vi "AutoTuneLockin.vi"() -> ()   [LabVIEW 2011]
panel:
  out "LockinXrange":dbl
  out "SlideY":cluster{dbl, dbl}(slide)={0.0, -1.6336633663366336} scale=-1.0..1.0
  out "Slide 2":cluster{dbl, dbl}(slide)={0.0, -1.6336633663366336} scale=-1.0..1.0
  out "Y":dbl
  out "X":dbl
  in  "stop":bool
  in  "Lockin":refnum<visa-resource-name>
  in  "Sr 830 sensitivity":T1(ring)
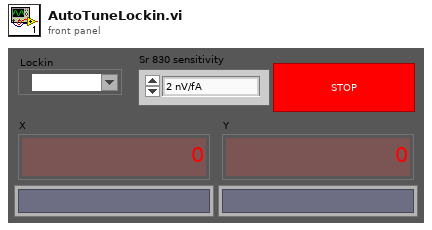
[diagram p1: front panel]
types:
  T1 = enum16{"2 nV/fA", "5 nV/fA", "10 nV/fA", "20 nV/fA", "50 nV/fA", "100 nV/fA", "200 nV/fA", "500 nV/fA", "1 uV/pA", "2 uV/pA", "5 uV/pA", "10 uV/pA", "20 uV/pA", "50 uV/pA", "100 uV/pA", "200 uV/pA", "500 uV/pA", "1 mV/nA", "2 mV/nA", "5 mV/nA", "10 mV/nA", "20 mV/nA", "50 mV/nA", "100 mV/nA", "200 mV/nA", "500 mV/nA", "1 V/uA"}
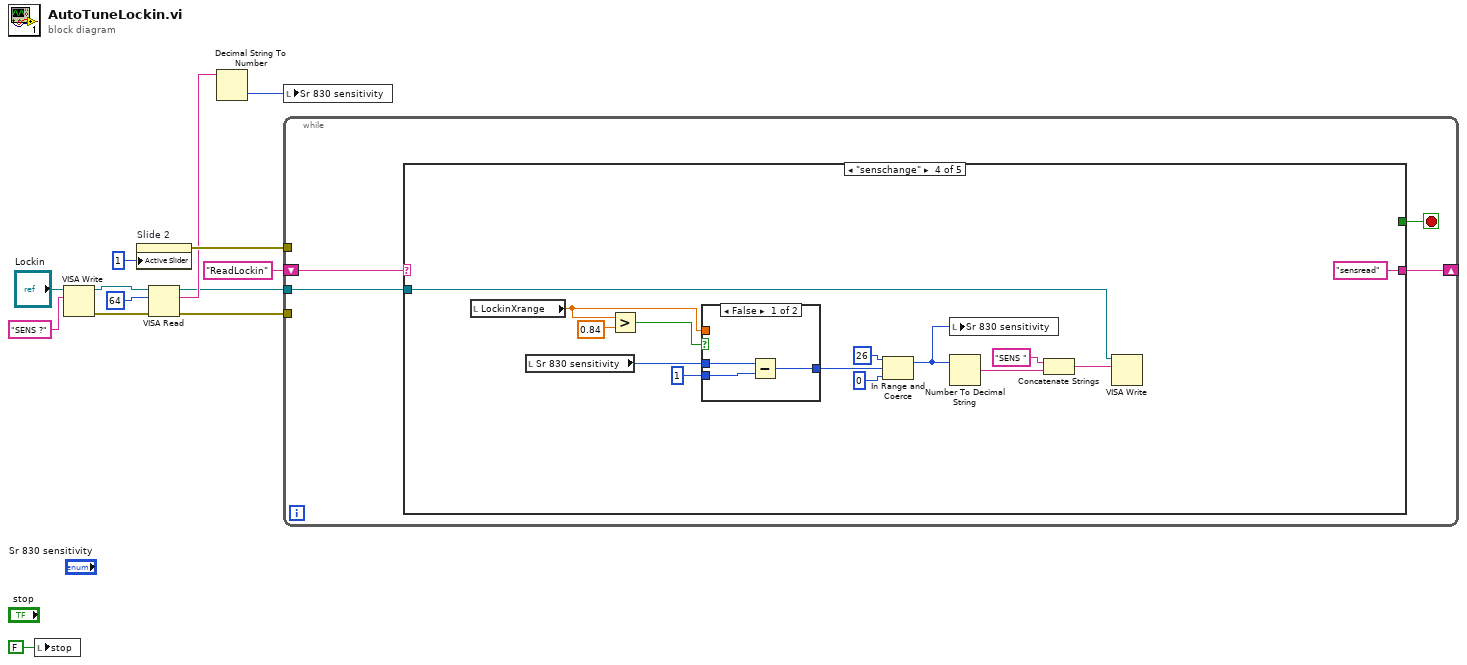
[diagram p0: block diagram]
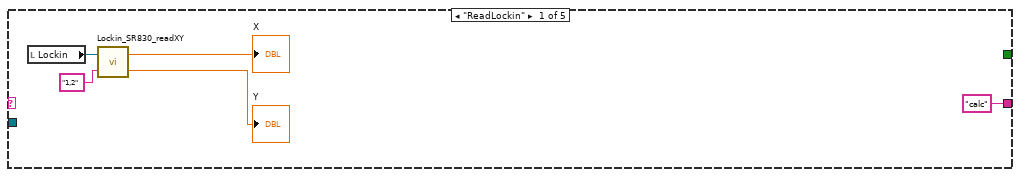
[diagram p2: hidden frame]
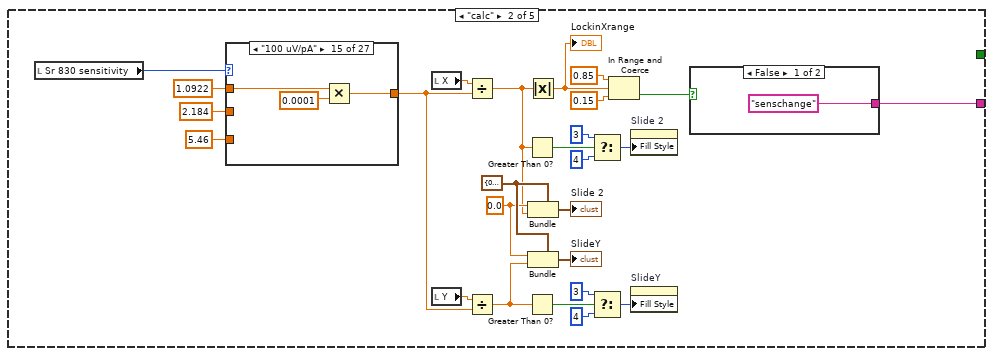
[diagram p3: hidden frame]
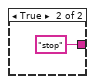
[diagram p4: hidden frame]
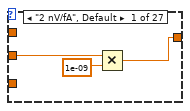
[diagram p5: hidden frame]
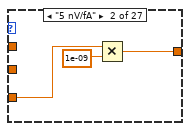
[diagram p6: hidden frame]
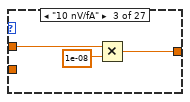
[diagram p7: hidden frame]
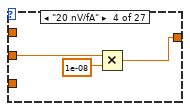
[diagram p8: hidden frame]
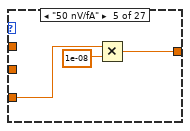
[diagram p9: hidden frame]
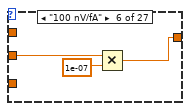
[diagram p10: hidden frame]
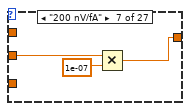
[diagram p11: hidden frame]
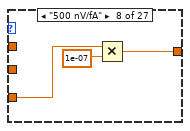
[diagram p12: hidden frame]
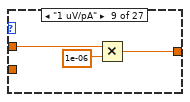
[diagram p13: hidden frame]
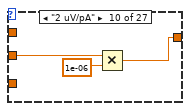
[diagram p14: hidden frame]
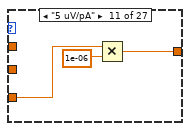
[diagram p15: hidden frame]
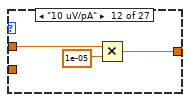
[diagram p16: hidden frame]
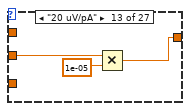
[diagram p17: hidden frame]
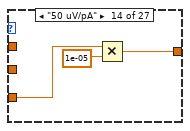
[diagram p18: hidden frame]
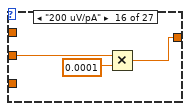
[diagram p19: hidden frame]
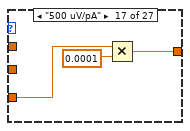
[diagram p20: hidden frame]
diagram:
  n1 = local write "stop"(FALSE ("stop")) -> ()
  n2 = VISA Write(VISA resource name="Lockin", write buffer="SENS ?" ("Command")) -> (VISA resource name out=w3:refnum<visa-resource-name>, error out=w6:errorcluster)  [unwired: 1 in, 1 out]
  n3 = property on="Slide 2" class="Slide (strict)"("Active Slider"=1) -> (error out=w11:errorcluster)  [unwired: 2 in, 1 out]
  n4 = VISA Read(VISA resource name=w3, byte count=u32 64 ("nombre d'octets"), error in (no error)=w6) -> (VISA resource name out=w1:refnum<visa-resource-name>, read buffer=w8:string, error out=w4:errorcluster)  [unwired: 1 out]
  n5 = Decimal String To Number(string=w8) -> (number=w9:i32)  [unwired: 2 in, 1 out]
  n6 = local write "Sr 830 sensitivity"(w9) -> ()
  n7 = while {
    shift-right: [w15] -> _
    shift-left: "ReadLockin" -> [w17]
    tunnel: w1 -> [w14]
    tunnel: w11 -> [_]
    tunnel: w4 -> [_]
    stop <- w16 stop-if-true
    n8 = case shown="\"senschange\"" w17 {
      tunnel: [_ _ _ _ w159] -> w16
      tunnel: ["calc" w24 "ReadLockin" "sensread" "ReadLockin"] -> w15
      tunnel: w14 -> [_ _ w132 w147 _]
      frame "ReadLockin" {
        n9 = local read "Lockin"() -> (w22:refnum<visa-resource-name>)
        n10 = call "Lockin_SR830_readXY.vi"("Variable"="1,2", "VISA Resource Name"=w22) -> ("Output Y"=→"Y":dbl, "Output X"=→"X":dbl)
      }
      frame "calc" {
        w36 = cluster{dbl, dbl} {0.0, 0.0} ("Slide")
        w34 = 0.0
        n11 = local read "Sr 830 sensitivity"() -> (w48:T1)
        n12 = case shown="\"100 uV/pA\"" w48 {
          tunnel: 1.0922 -> [_ _ w58 _ _ _ _ _ w76 _ _ w85 _ _ w94 _ _ w103 _ _ w112 _ _ w121 _ _ w129]
          tunnel: [w51 w54 w57 w60 w63 w66 w69 w72 w75 w78 w81 w84 w87 w90 w93 w96 w99 w102 w105 w108 w111 w114 w117 w120 w123 w126 w129] -> w42
          tunnel: 2.184 -> [w52 _ _ w61 _ w67 w70 _ _ w80 _ _ w88 _ _ w97 _ _ w106 _ _ w115 _ _ w124 _ _]
          tunnel: 5.46 -> [_ w55 _ _ w64 _ _ w73 _ _ w82 _ _ w91 _ _ w100 _ _ w109 _ _ w118 _ _ w127 _]
          frame "2 nV/fA", Default {
            n13 = Multiply(x=w52, y=1e-09) -> (x*y=w51:dbl)
          }
          frame "5 nV/fA" {
            n14 = Multiply(x=w55, y=1e-09) -> (x*y=w54:dbl)
          }
          frame "10 nV/fA" {
            n15 = Multiply(x=w58, y=1e-08) -> (x*y=w57:dbl)
          }
          frame "20 nV/fA" {
            n16 = Multiply(x=w61, y=1e-08) -> (x*y=w60:dbl)
          }
          frame "50 nV/fA" {
            n17 = Multiply(x=w64, y=1e-08) -> (x*y=w63:dbl)
          }
          frame "100 nV/fA" {
            n18 = Multiply(x=w67, y=1e-07) -> (x*y=w66:dbl)
          }
          frame "200 nV/fA" {
            n19 = Multiply(x=w70, y=1e-07) -> (x*y=w69:dbl)
          }
          frame "500 nV/fA" {
            n20 = Multiply(x=w73, y=1e-07) -> (x*y=w72:dbl)
          }
          frame "1 uV/pA" {
            n21 = Multiply(x=w76, y=1e-06) -> (x*y=w75:dbl)
          }
          frame "2 uV/pA" {
            n22 = Multiply(x=w80, y=1e-06) -> (x*y=w78:dbl)
          }
          frame "5 uV/pA" {
            n23 = Multiply(x=w82, y=1e-06) -> (x*y=w81:dbl)
          }
          frame "10 uV/pA" {
            n24 = Multiply(x=w85, y=1e-05) -> (x*y=w84:dbl)
          }
          frame "20 uV/pA" {
            n25 = Multiply(x=w88, y=1e-05) -> (x*y=w87:dbl)
          }
          frame "50 uV/pA" {
            n26 = Multiply(x=w91, y=1e-05) -> (x*y=w90:dbl)
          }
          frame "100 uV/pA" {
            n27 = Multiply(x=w94, y=0.0001) -> (x*y=w93:dbl)
          }
          frame "200 uV/pA" {
            n28 = Multiply(x=w97, y=0.0001) -> (x*y=w96:dbl)
          }
          frame "500 uV/pA" {
            n29 = Multiply(x=w100, y=0.0001) -> (x*y=w99:dbl)
          }
          frame "1 mV/nA" {
            n30 = Multiply(x=w103, y=0.001) -> (x*y=w102:dbl)
          }
          frame "2 mV/nA" {
            n31 = Multiply(x=w106, y=0.001) -> (x*y=w105:dbl)
          }
          frame "5 mV/nA" {
            n32 = Multiply(x=w109, y=0.001) -> (x*y=w108:dbl)
          }
          frame "10 mV/nA" {
            n33 = Multiply(x=w112, y=0.01) -> (x*y=w111:dbl)
          }
          frame "20 mV/nA" {
            n34 = Multiply(x=w115, y=0.01) -> (x*y=w114:dbl)
          }
          frame "50 mV/nA" {
            n35 = Multiply(x=w118, y=0.01) -> (x*y=w117:dbl)
          }
          frame "100 mV/nA" {
            n36 = Multiply(x=w121, y=0.1) -> (x*y=w120:dbl)
          }
          frame "200 mV/nA" {
            n37 = Multiply(x=w124, y=0.1) -> (x*y=w123:dbl)
          }
          frame "500 mV/nA" {
            n38 = Multiply(x=w127, y=0.1) -> (x*y=w126:dbl)
          }
          frame "1 V/uA" {
          }
        }
        n39 = local read "X"() -> (w44:dbl)
        n40 = local read "Y"() -> (w43:dbl)
        n41 = Divide(x=w44, y=w42) -> (x/y=w28:dbl)
        n42 = Divide(x=w43, y=w42) -> (x/y=w30:dbl)
        n43 = Greater Than 0?(x=w28) -> (x > 0?=w41:bool)
        n44 = Greater Than 0?(x=w30) -> (x > 0?=w33:bool)
        n45 = Absolute Value(x=w28) -> (abs(x)=w23:dbl)
        "LockinXrange" <- w23
        n46 = Bundle(cluster=w36, w34, w28) -> (→"Slide 2":cluster{dbl, dbl})
        n47 = Bundle(cluster=w36, w34, w30) -> (→"SlideY":cluster{dbl, dbl})
        n48 = Select(t=3 ("Fill Style"), s=w41, f=4 ("Fill Style")) -> (s? t:f=w37:i32)
        n49 = Select(t=3 ("Fill Style"), s=w33, f=4 ("Fill Style")) -> (s? t:f=w29:i32)
        n50 = In Range and Coerce(upper limit=0.85, x=w23, lower limit=0.15 ("upper limit")) -> (In Range?=w25:bool)  [unwired: 1 out]
        n51 = property on="Slide 2" class="Slide (strict)"("Fill Style"=w37) -> ()  [unwired: 2 in, 2 out]
        n52 = property on="SlideY" class="Slide (strict)"("Fill Style"=w29) -> ()  [unwired: 2 in, 2 out]
        n53 = case shown="False" w25 {
          tunnel: ["senschange" "stop"] -> w24
          frame False {
          }
          frame True {
          }
        }
      }
      frame "sensread" {
        n54 = VISA Write(VISA resource name=w132, write buffer="SENS ?" ("Command")) -> (VISA resource name out=w136:refnum<visa-resource-name>, error out=w135:errorcluster)  [unwired: 1 in, 1 out]
        n55 = VISA Read(VISA resource name=w136, byte count=u32 64 ("nombre d'octets"), error in (no error)=w135) -> (read buffer=w133:string)  [unwired: 3 out]
        n56 = Decimal String To Number(string=w133) -> (number=w130:i32)  [unwired: 2 in, 1 out]
        n57 = local write "Sr 830 sensitivity"(w130) -> ()
      }
      frame "senschange" {
        n58 = local read "LockinXrange"() -> (w143:dbl)
        n59 = local read "Sr 830 sensitivity"() -> (w144:T1)
        n60 = Greater?(x=w143, y=0.84) -> (0:w145:bool)
        n61 = case shown="False" w145 {
          tunnel: w144 -> [w154 w157]
          tunnel: w143 -> [_ _]
          tunnel: 1 ("y") -> [w153 w156]
          tunnel: [w152 w155] -> w141
          frame False {
            n62 = Subtract(x=w154, y=w153) -> (x-y=w152:i32)
          }
          frame True {
            n63 = Add(x=w157, y=w156) -> (x+y=w155:i32)
          }
        }
        n64 = In Range and Coerce(upper limit=26, x=w141, lower limit=0) -> (coerced(x)=w138:i32)  [unwired: 1 out]
        n65 = local write "Sr 830 sensitivity"(w138) -> ()
        n66 = Number To Decimal String(number=w138) -> (decimal integer string=w150:string)  [unwired: 1 in]
        n67 = Concatenate Strings("SENS " ("chaîne"), w150) -> (w148:string)
        n68 = VISA Write(VISA resource name=w147, write buffer=w148) -> ()  [unwired: 1 in, 3 out]
      }
      frame "stop", Default {
        n69 = Wait (ms)(milliseconds to wait=u32 6173) -> ()  [unwired: 1 out]
        n70 = local read "stop"() -> (w158:bool)
        n71 = flat-sequence {
          tunnel: [w162] -> w159
          tunnel: w158 -> [w162]
          frame #0 {
          }
        }
      }
    }
  }
